vi "list rt targets.vi"() -> (3 "desktop targets":T1[](array[typedef]))   [LabVIEW 2013, in "TBM configuration.lvclass"]
uses:
  TBM configuration.lvclass
  Target Types.ctl
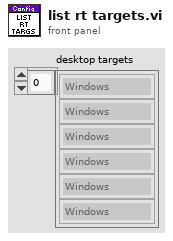
[diagram p1: front panel]
types:
  T1 = typedef "TBM configuration.lvclass/Target Types.ctl" = enum16{"Windows", "Mac", "Linux", "Linux RT ARM", "VxWorks", "Pharlap", "Other", "Linux RT x64"}
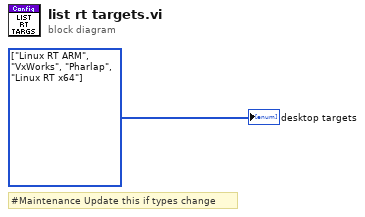
[diagram p0: block diagram]
diagram:
  w1 = T1[] [enum."Linux RT ARM", enum."VxWorks", enum."Pharlap", enum."Linux RT x64"] items=["Windows", "Mac", "Linux", "Linux RT ARM", "VxWorks", "Pharlap", "Other", "Linux RT x64"] ("desktop targets")
  # "#Maintenance Update this if types change"
  "desktop targets" <- w1
